vi "AverageOneCoord(SubVI).vi"(0 "Array":dbl[](array[numeric]), 9 "Number of pins":i32=5, 11 "Number of images each":i32=10) -> (4 "Averages":dbl[][](array[numeric]), 8 "SD":dbl[][](array[numeric]))   [LabVIEW 2017]
uses:
  <vilib>/Analysis/NI_AALBase.lvlib
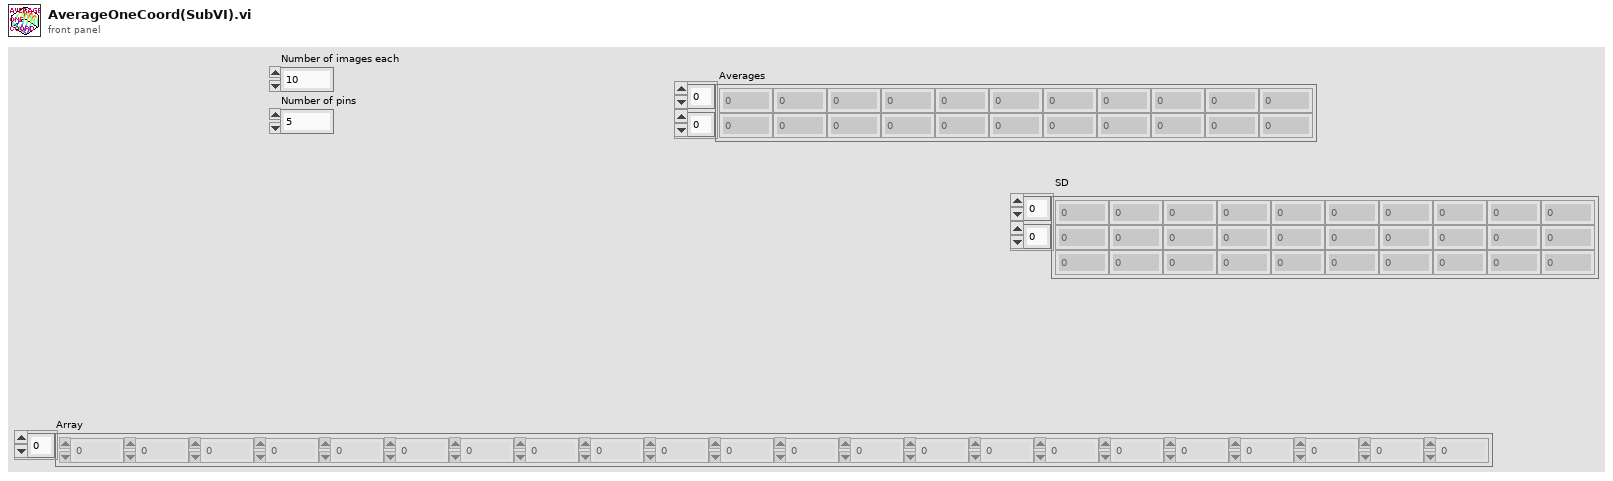
[diagram p1: front panel]
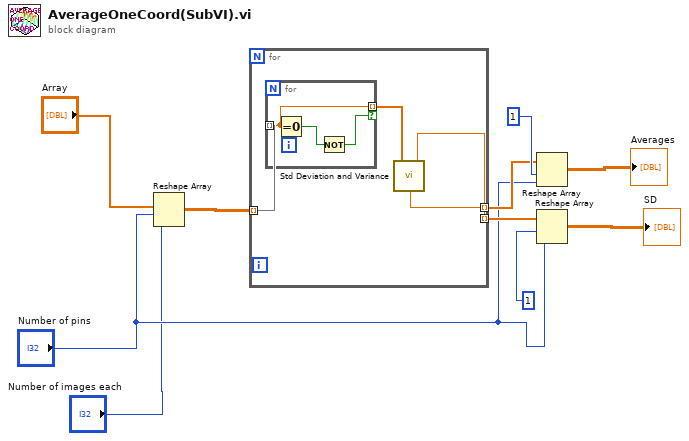
[diagram p0: block diagram]
diagram:
  n1 = Reshape Array("Array", "Number of pins", "Number of images each") -> (w10:dbl[][])
  n2 = for {
    tunnel: w10 -> [w11] mode=indexing
    tunnel: [w14] -> w6 mode=indexing
    tunnel: [w13] -> w5 mode=indexing
    n3 = for {
      tunnel: w11 -> [w17] mode=indexing
      tunnel: [w17] -> w12 mode=indexing if=w15
      n4 = Equal To 0?(x=w17) -> (x = 0?=w16:bool)
      n5 = Not(x=w16) -> (.not. x?=w15:bool)
    }
    n6 = call <vilib>:"Std Deviation and Variance.vi"("X"=w12) -> ("mean"=w14:dbl, "standard deviation"=w13:dbl)  [unwired: 1 in, 1 out]
  }
  n7 = Reshape Array(w6, 1 ("dimension size"), "Number of pins") -> (→"Averages":dbl[][])
  n8 = Reshape Array(w5, 1 ("dimension size"), "Number of pins") -> (→"SD":dbl[][])
